vi "Essalihi_Youssef-projet-Acquisition-Donnees.vi"() -> ()   [LabVIEW 2022 SP3]
uses:
  <vilib>/Utility/sysdir.llb/System Directory Type.ctl
  <vilib>/Utility/file.llb/Write Delimited Spreadsheet (DBL).vi
panel:
  out "Temperature_Display":dbl[][](graph)
  in  "Emergency_Stop":bool
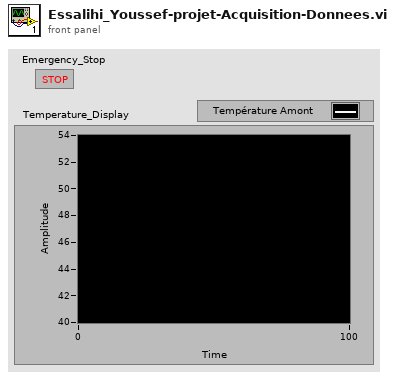
[diagram p1: front panel]
types:
  T1 = typedef "System Directory Type.ctl" = i32
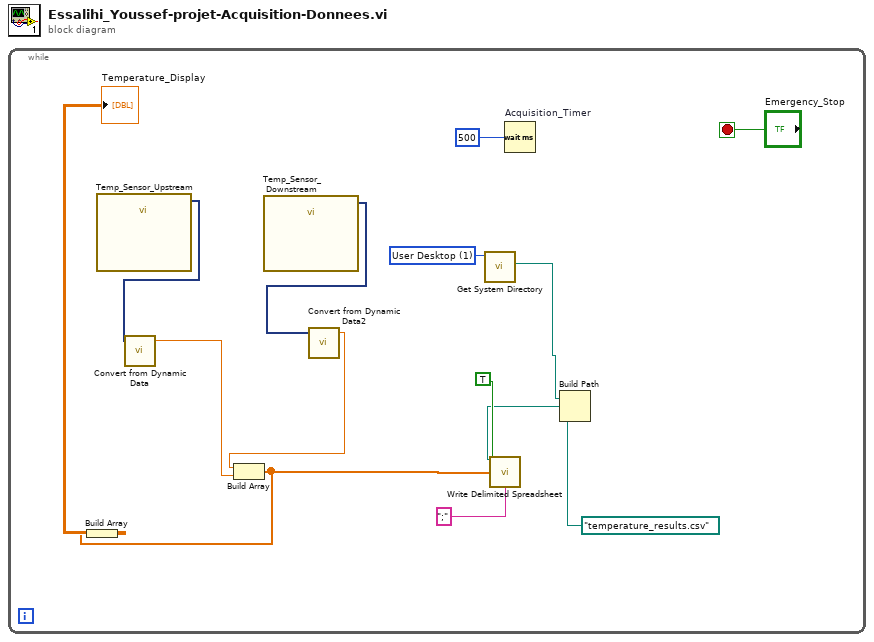
[diagram p0: block diagram]
diagram:
  n1 = while {
    stop <- "Emergency_Stop" stop-if-true
    w1 = T1 1 items=["User Home"=0, "User Desktop"=1, "User Documents"=2, "User Application Data"=3, "User Preferences"=4, "User Temporary"=5, "Public Documents"=6, "Public Application Data"=7, "Public Preferences"=8, "Public Cache"=13, "System Core Libraries"=9, "System Installed Libraries"=10, "Application Files"=11, "Boot Volume Root"=12] ("system directory type")
    n2 = call "Temp_Sensor_Upstream"() -> ("Sine"=w12:dynamicdata)  [unwired: 14 in, 1 out]
    n3 = call "Convert from Dynamic Data"("Dynamic Data Type"=w12) -> ("Scalar"=w8:dbl)  [unwired: 3 in]
    n4 = call "Temp_Sensor_Downstream"() -> ("Sine"=w11:dynamicdata)  [unwired: 14 in, 1 out]
    n5 = call "Convert from Dynamic Data2"("Dynamic Data Type"=w11) -> ("Scalar"=w9:dbl)  [unwired: 3 in]
    n6 = Build Array(w9, w8) -> (w7:dbl[])
    n7 = Build Array(w7) -> (→"Temperature_Display":dbl[][])
    n8 = call <vilib>:"Get System Directory.vi"("system directory type"=w1) -> ("system directory"=w2:path)  [unwired: 10 in]
    n9 = Wait (ms) "Acquisition_Timer"(milliseconds to wait=u32 500) -> ()  [unwired: 1 out]
    n10 = Build Path(base path=w2, name or relative path=path "temperature_results.csv") -> (appended path=w3:path)
    n11 = call-poly <vilib>:"Write Delimited Spreadsheet.vi"("file path (dialog if empty)"=w3, "1D data"=w7, "append to file? (new file:F)"=TRUE, "delimiter (\\t)"=";" ("delimiter (\\t)")) -> ()  [unwired: 10 in, 2 out]
  }
